vi "NPL_Simulated Temperature Control.vi"() -> ()   [LabVIEW 2011]
panel:
  in  "TCP port":u16=12344
  in  "error in (no error)":errorcluster
  out "error out":errorcluster
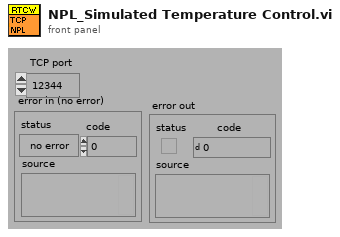
[diagram p1: front panel]
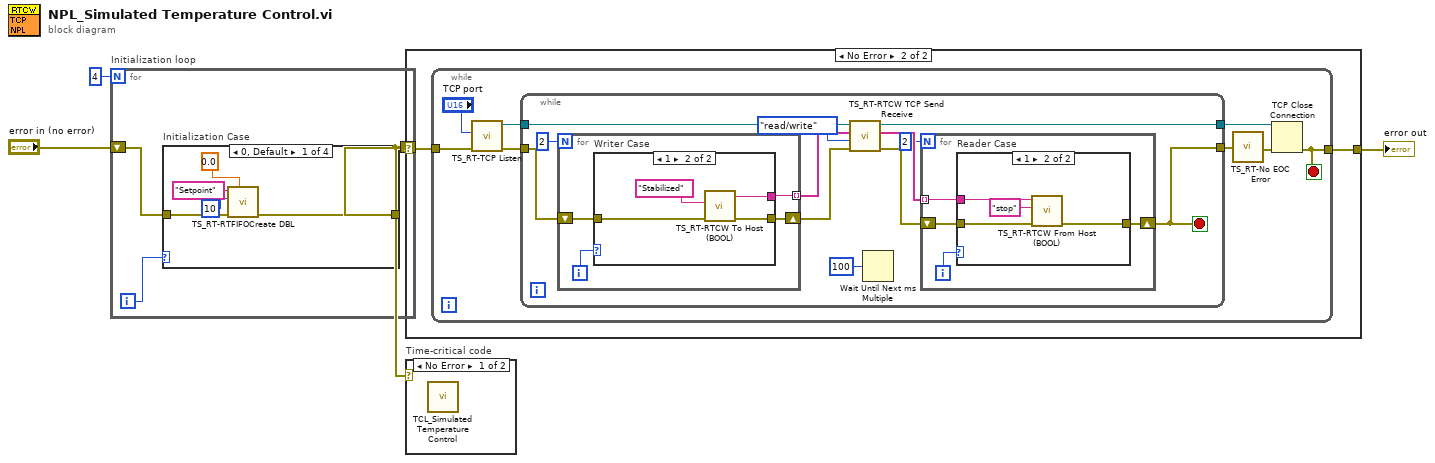
[diagram p0: block diagram]
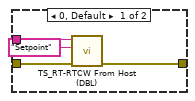
[diagram p4: hidden frame]
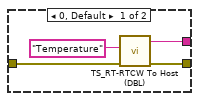
[diagram p5: hidden frame]
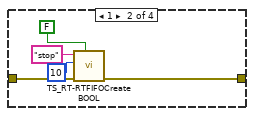
[diagram p6: hidden frame]
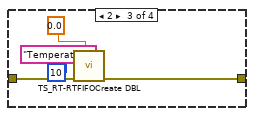
[diagram p7: hidden frame]
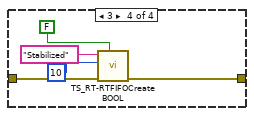
[diagram p8: hidden frame]
diagram:
  n1 = for "Initialization loop" {
    N: 4 -> [_]
    shift-right: [w5] -> w2
    shift-left: "error in (no error)" -> [w6]
    i -> [w7]
    n2 = case "Initialization Case" shown="0, Default" w7 {
      tunnel: w6 -> [w12 w17 w22 w27]
      tunnel: [w11 w16 w21 w26] -> w5
      frame 0, Default {
        n3 = call "TS_RT-RTFIFOCreate DBL.vi"("type"=0.0, "error in (no error)"=w12, "size (10)"=u32 10, "name (unnamed)"="Setpoint") -> ("error out"=w11:errorcluster)  [unwired: 1 in, 6 out]
      }
      frame 1 {
        n4 = call "TS_RT-RTFIFOCreate BOOL.vi"("type"=FALSE, "error in (no error)"=w17, "size (10)"=u32 10, "name (unnamed)"="stop") -> ("error out"=w16:errorcluster)  [unwired: 1 in, 6 out]
      }
      frame 2 {
        n5 = call "TS_RT-RTFIFOCreate DBL.vi"("type"=0.0, "error in (no error)"=w22, "size (10)"=u32 10, "name (unnamed)"="Temperature") -> ("error out"=w21:errorcluster)  [unwired: 1 in, 6 out]
      }
      frame 3 {
        n6 = call "TS_RT-RTFIFOCreate BOOL.vi"("type"=FALSE, "error in (no error)"=w27, "size (10)"=u32 10, "name (unnamed)"="Stabilized") -> ("error out"=w26:errorcluster)  [unwired: 1 in, 6 out]
      }
    }
  }
  n7 = case shown="No Error" w2 {
    selector: w2 -> [w28 w29]
    tunnel: [w28 w30] -> w4
    frame Error {
    }
    frame No Error {
      n8 = while "While Loop1" {
        tunnel: [w35] -> w30
        tunnel: w29 -> [w33]
        stop <- w35 stop-if-true
        n9 = call "TS_RT-TCP Listen.vi"("error in (no error)"=w33, "port"="TCP port") -> ("error out"=w32:errorcluster, "connection ID"=w36:refnum<k5>)  [unwired: 1 in, 7 out]
        n10 = while "While Loop2" {
          tunnel: w36 -> [w50]
          tunnel: [w49] -> w37
          tunnel: w32 -> [w46]
          tunnel: [w44] -> w31
          stop <- w44 stop-if-true
          n11 = for {
            N: 2 -> [_]
            tunnel: [w66] -> w47 mode=indexing
            shift-right: [w63] -> w45
            shift-left: w46 -> [w64]
            i -> [w65]
            n12 = case "Writer Case" shown="1" w65 {
              tunnel: [w68 w72] -> w66
              tunnel: [w69 w73] -> w63
              tunnel: w64 -> [w70 w74]
              frame 0, Default {
                n13 = call "TS_RT-RTCW To Host (DBL).vi"("error in (no error)"=w70, "name (unnamed)"="Temperature") -> ("error out"=w69:errorcluster, "Data"=w68:string)  [unwired: 8 out]
              }
              frame 1 {
                n14 = call "TS_RT-RTCW To Host (BOOL).vi"("error in (no error)"=w74, "name (unnamed)"="Stabilized") -> ("error out"=w73:errorcluster, "Data"=w72:string)  [unwired: 8 out]
              }
            }
          }
          n15 = call "TS_RT-RTCW TCP Send Receive.vi"("error in (no error)"=w45, "access (read/write)"=enum16{"read/write", "read only", "write only"}."read/write", "Data In"=w47, "connection ID"=w50) -> ("error out"=w43:errorcluster, "Data Out"=w48:string[], "connection ID Out"=w49:refnum<k5>)  [unwired: 1 out]
          n16 = Wait Until Next ms Multiple(millisecond multiple=u32 100) -> ()  [unwired: 1 out]
          n17 = for {
            N: 2 -> [_]
            tunnel: w48 -> [w53] mode=indexing
            shift-right: [w52] -> w44
            shift-left: w43 -> [w51]
            i -> [w54]
            n18 = case "Reader Case" shown="1" w54 {
              tunnel: w51 -> [w57 w61]
              tunnel: [w58 w62] -> w52
              tunnel: w53 -> [w56 w60]
              frame 0, Default {
                n19 = call "TS_RT-RTCW From Host (DBL).vi"("error in"=w57, "name (unnamed)"="Setpoint", "Data In"=w56) -> ("error out"=w58:errorcluster)  [unwired: 8 out]
              }
              frame 1 {
                n20 = call "TS_RT-RTCW From Host (BOOL).vi"("error in"=w61, "name (unnamed)"="stop", "Data In"=w60) -> ("error out"=w62:errorcluster)  [unwired: 8 out]
              }
            }
          }
        }
        n21 = call "TS_RT-No EOC Error.vi"("error in (no error)"=w31) -> ("error out"=w38:errorcluster)  [unwired: 4 out]
        n22 = TCP Close Connection(connection ID=w37, error in (no error)=w38) -> (error out=w35:errorcluster)  [unwired: 2 out]
      }
    }
  }
  "error out" <- w4
  n23 = case "Time-critical code" shown="No Error" w2 {
    frame No Error {
      n24 = call "TCL_Simulated Temperature Control.vi"() -> ()  [unwired: 1 out]
    }
    frame Error {
    }
  }
